vi "LibXML_GetAttributeNameAndValue.vi"(8 "error in":errorcluster, 10 "attribute":u32) -> (0 "error out":errorcluster, 2 "value":string, 3 "name":string)   [LabVIEW 2019, in "Tools.lvlib" / "LibXML.lvlib"]
doc: "Gets the name and value strings of the attribute (U32) input."
uses:
  LibXML.lvlib
  LibXML_NavigateDirection.ctl
  LibXML_GetNodeStrPtr.vi
  LibXML_GetNodeResolvedContentStrPointer.vi
  LibXML_GetStringLength.vi
  LibXML_CopyString.vi
  Error Cluster From Error Code_subroutine.vi
  <vilib>/Utility/error.llb/Trim Whitespace.vi
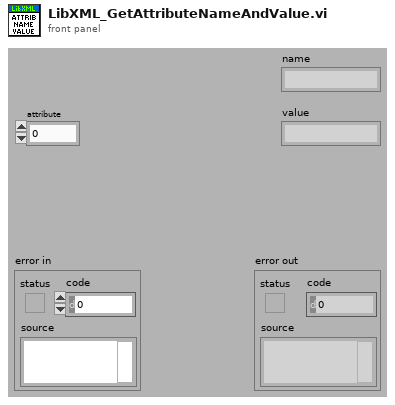
[diagram p1: front panel]
types:
  T1 = typedef "Tools.lvlib/LibXML.lvlib/LibXML_NavigateDirection.ctl" = enum16{"NOP", "first child", "last child", "parent", "next", "prev"}
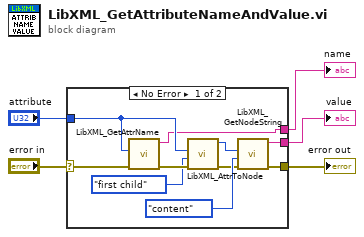
[diagram p0: block diagram]
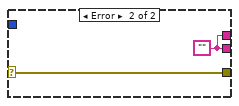
[diagram p2: hidden frame]
diagram:
  n1 = case shown="No Error" "error in" {
    selector: "error in" -> [w10 w17]
    tunnel: [w9 w17] -> w4
    tunnel: "attribute" -> [w8 _]
    tunnel: [w7 w16] -> w2
    tunnel: [w6 w16] -> w1
    frame No Error {
      n2 = call "LibXML_GetAttrName.vi"("error in"=w10, "attribute"=w8) -> ("error out"=w14:errorcluster, "lvstring"=w7:string)  [unwired: 8 in]
      n3 = call "LibXML_AttrToNode.vi"("error in"=w14, "direction"=LibXML_NavigateDirection."first child", "attribute in"=w8) -> ("error out"=w13:errorcluster, "node out"=w12:u32)  [unwired: 7 in]
      n4 = call "LibXML_GetNodeString.vi"("error in"=w13, "type"=enum16{"NOP", "name", "content"}."content", "node"=w12) -> ("error out"=w9:errorcluster, "lvstring"=w6:string)  [unwired: 7 in]
    }
    frame Error {
      w16 = ""
    }
  }
  "error out" <- w4
  "name" <- w2
  "value" <- w1
